vi "instance count allowed.vi"(8 "error in":errorcluster, 11 "ExampleSequencer configuration in":refnum<class "ExampleSequencer configuration.lvclass">) -> (0 "error out":errorcluster, 2 "instances allowed":i32, 3 "ExampleSequencer configuration out":refnum<class "ExampleSequencer configuration.lvclass">)   [LabVIEW 2017, in "ExampleSequencer configuration.lvclass"]
uses:
  ExampleSequencer configuration.lvclass
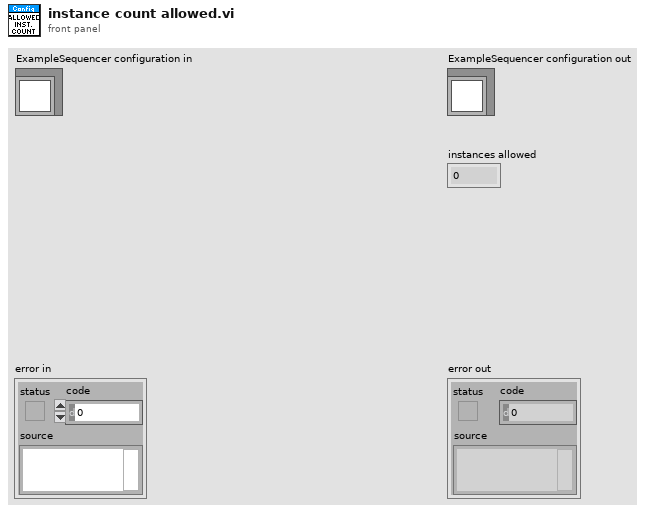
[diagram p1: front panel]
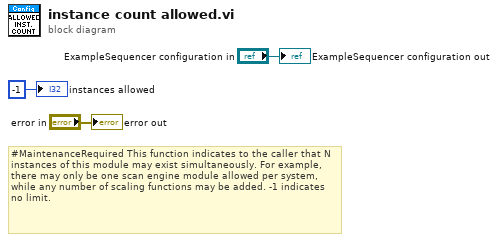
[diagram p0: block diagram]
diagram:
  # "#MaintenanceRequired This function indicates to the caller that N instances of this module may exist simultaneously. For example, there may only be one scan engine module allowed per system, while any number of scaling functions may be added. -1 indicates no limit."
  "error out" <- "error in"
  "ExampleSequencer configuration out" <- "ExampleSequencer configuration in"
  "instances allowed" <- -1 ("instances allowed")
